vi "Get Field Config.vi"(8 "error in (no error)":errorcluster, 11 "Ctrl Refnum Column in":refnum<class "Ctrl Refnum Column.lvclass">) -> (0 "error out":errorcluster, 2 "Field Config":refnum<class "Field Configuration.lvclass">, 3 "Ctrl Refnum Column out":refnum<class "Ctrl Refnum Column.lvclass">)   [LabVIEW 2020, in "Basic Fields.lvlib" / "Ctrl Refnum Column.lvclass"]
uses:
  Ctrl Refnum Column.lvclass
  Field Interfaces/Field Configuration Interface Class/Field Configuration.lvclass
  Ctrl Refnum Column.lvclass/Ctrl Refnum Column.ctl
  Basic Columns/Basic Columns/Column Class/Column Parent.lvclass
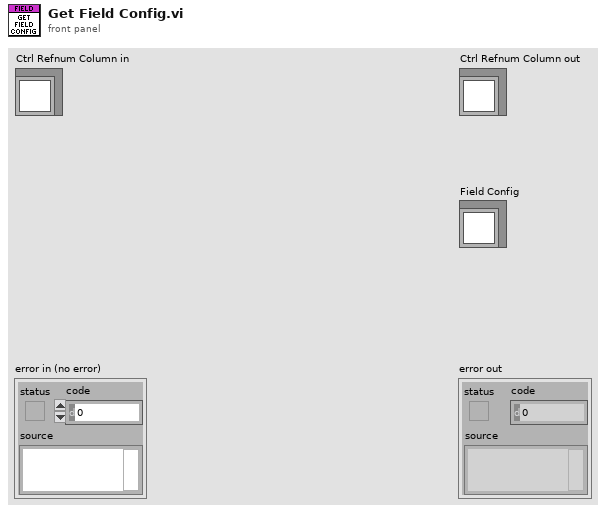
[diagram p1: front panel]
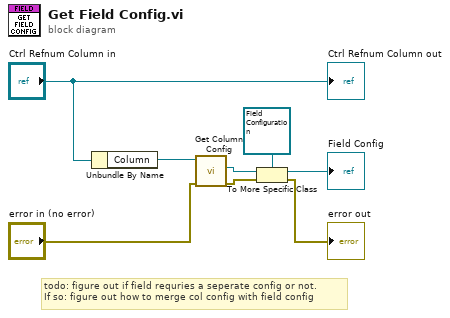
[diagram p0: block diagram]
diagram:
  # "todo: figure out if field requries a seperate config or not.\nIf so: figure out how to merge col config with field config"
  n1 = Unbundle By Name("Ctrl Refnum Column in") -> ("Column"=w7:refnum<class "Column Parent.lvclass">)
  n2 = call-dynamic "Get Column Config.vi"("error in (no error)"="error in (no error)", "Column Parent in"=w7) -> ("error out"=w4:errorcluster, "Column Configuration"=w5:refnum<class "Column Configuration.lvclass">)  [unwired: 7 in, 1 out]
  n3 = To More Specific Class(target class=refnum<class "Field Configuration.lvclass"> refnum ("Field Interfaces.lvlib:Field Configuration.lvclass"), reference=w5, error in=w4) -> (specific class reference=→"Field Config":refnum<class "Field Configuration.lvclass">, error out=→"error out":errorcluster)
  "Ctrl Refnum Column out" <- "Ctrl Refnum Column in"
